vi "StatusUpdate.vi"(8 "error in (no error)":errorcluster, 9 "Status":string, 11 "Module":refnum<class "ModuleAdmin.lvclass">) -> (0 "error out":errorcluster, 3 "Module":refnum<class "ModuleAdmin.lvclass">)   [LabVIEW 2018, in "MyPlugins.lvlib"]
doc: "Sends a message from the module indicating the status of the prior request."
uses:
  MyPlugins.lvlib
  <userlib>/NIST/ModuleAdminLib/ModuleAdmin/ModuleAdmin.lvclass
  PluginsShared/clEventType.ctl
  PluginsShared/PluginsShared.lvlib
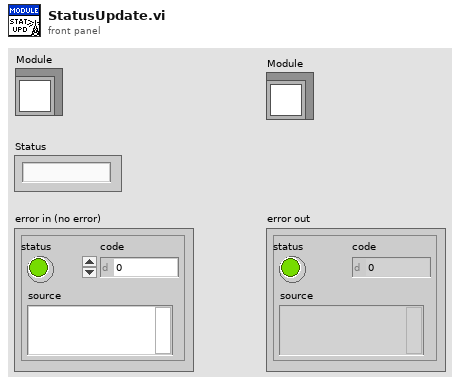
[diagram p1: front panel]
types:
  T1 = typedef "PluginsShared.lvlib/clEventType.ctl" = cluster{"ModuleID":i32, "Data":variant}
  T2 = typedef "PluginsShared.lvlib/clBroadcastEvents.ctl" = cluster{"DidInit":refnum<user-event>, "StatusUpdate":refnum<user-event>, "ErrorReport":refnum<user-event>, "DidStop":refnum<user-event>, "PathToINI":refnum<user-event>, "ReloadINIFiles":refnum<user-event>}
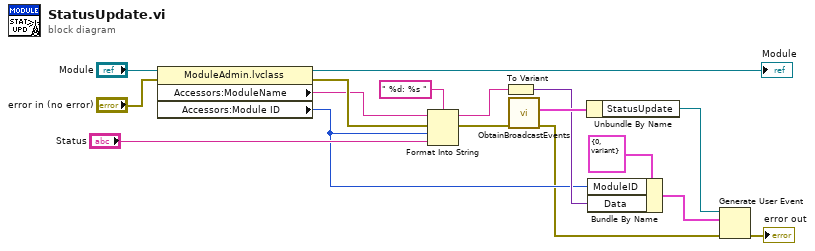
[diagram p0: block diagram]
diagram:
  n1 = property class="ModuleAdmin.lvclass"(reference="Module", error in="error in (no error)") -> (reference out=→"Module":refnum<class "ModuleAdmin.lvclass">, error out=w4:errorcluster, "Accessors:ModuleName"=w1:string, "Accessors:Module ID"=w7:i32)
  n2 = Format Into String(format string=" %d: %s ", initial string=w1, error in=w4, w7, "Status") -> (resulting string=w8:string, error out=w3:errorcluster)
  n3 = To Variant(anything=w8) -> (Variant=w14:variant)
  n4 = call "ObtainBroadcastEvents.vi"("error in (no error)"=w3) -> ("error out"=w2:errorcluster, "clBroadcastEvents"=w17:T2)  [unwired: 9 in]
  n5 = Unbundle By Name(w17) -> ("StatusUpdate"=w16:refnum<user-event>)
  n6 = Bundle By Name(cluster=T1 {"ModuleID"=0, "Data"=variant} ("clBroadcast"), "ModuleID"=w7, "Data"=w14) -> (w13:T1)
  n7 = Generate User Event(user event=w16, event data cluster=w13, error in=w2) -> (error out=→"error out":errorcluster)  [unwired: 1 in, 1 out]
